vi "Q8381 CURSOR ON-OFF.vi"(1 "off/ on":u16(ring) items=["CURSOR  OFF", "CURSOR  ON"], 2 "GPIB Address":u16=8 max=31 step=1, 3 "VISA resource name":refnum<visa-resource-name>) -> (0 "GPIB Status":bool)   [LabVIEW 2017]
doc: "off/on: 0: Cursor off, 1: Cursor on."
panel:
  out "Program Code":string
  # "CURSOR  ON/OFF"
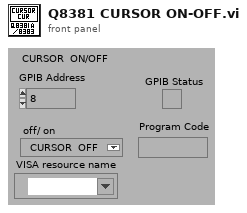
[diagram p1: front panel]
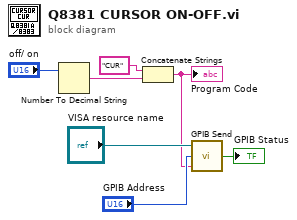
[diagram p0: block diagram]
diagram:
  n1 = Number To Decimal String(number="off/ on") -> (decimal integer string=w6:string)  [unwired: 1 in]
  n2 = Concatenate Strings("CUR", w6) -> (w2:string)
  "Program Code" <- w2
  n3 = call "GPIB Send.vi"("Command String"=w2, "Address"="GPIB Address", "VISA resource name"="VISA resource name") -> ("Error"=→"GPIB Status":bool)
